vi "Data Logger Open Config.vi"(8 "error in":errorcluster, 10 "Cluster":T1, 11 "Path":path) -> (0 "error out":errorcluster)   [LabVIEW 2014]
uses:
  TypeDef/Datalogger_State_OpenConfigFile.ctl
  <vilib>/Utility/config.llb/Read Key (String).vi
  <vilib>/Utility/config.llb/Read Key (U32).vi
  <vilib>/Utility/config.llb/Read Key (Path).vi
  <vilib>/Utility/config.llb/Read Key (Boolean).vi
  <vilib>/Utility/config.llb/NI_LVConfig.lvlib
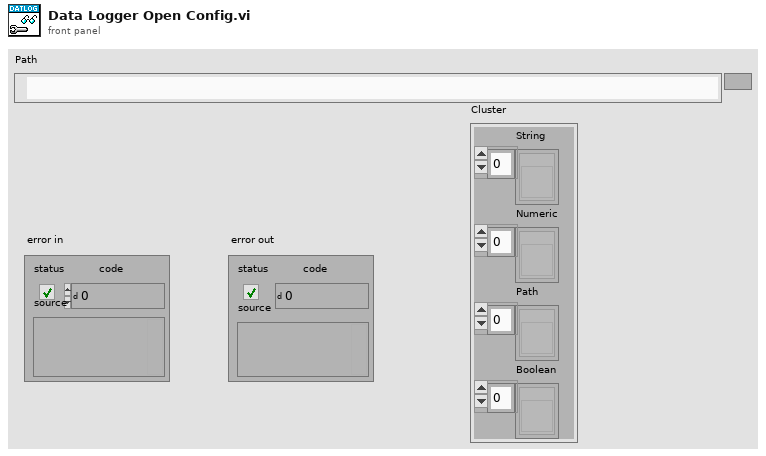
[diagram p1: front panel]
types:
  T1 = cluster{"String":refnum<vi>[], "Numeric":refnum<vi>[], "Path":refnum<vi>[], "Boolean":refnum<vi>[]}
  T2 = typedef "Datalogger_State_OpenConfigFile.ctl" = enum16{"Check config file?", "Open File", "Item 1", "Item 2", "Item 3", "Item 4", "Close File"}
  T3 = typedef "NI_LVConfig.lvlib/Config Data RefNum.ctl" = refnum<k1>
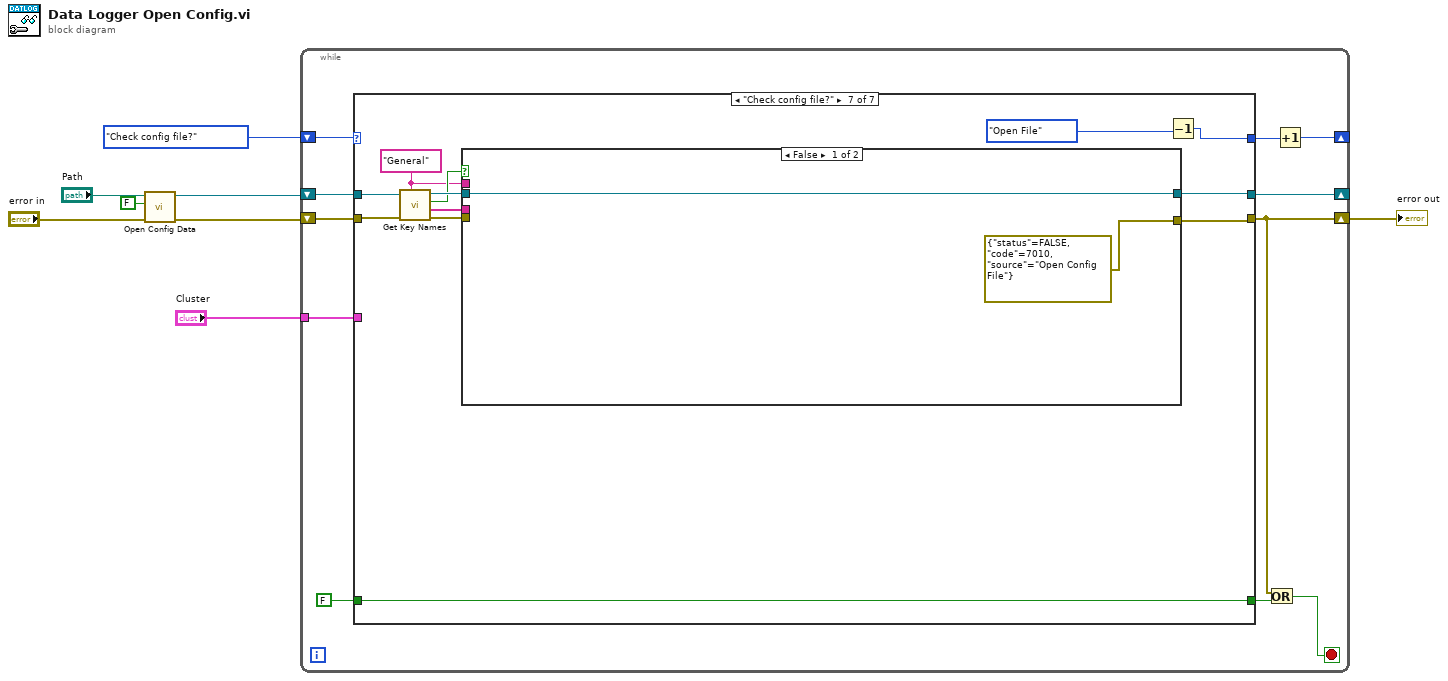
[diagram p0: block diagram]
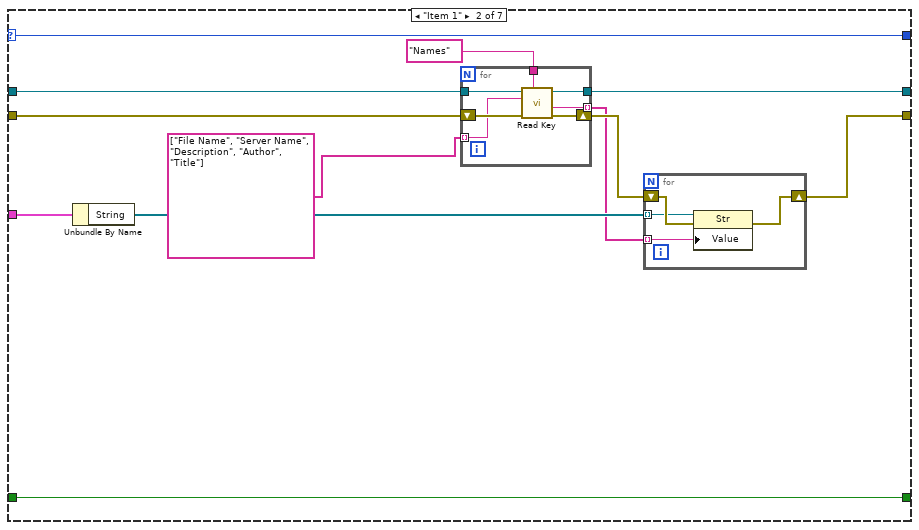
[diagram p3: hidden frame]
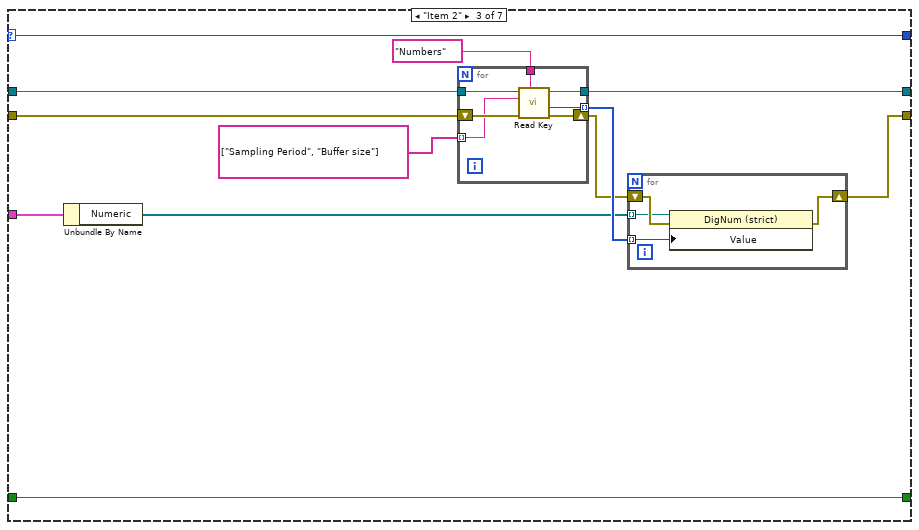
[diagram p4: hidden frame]
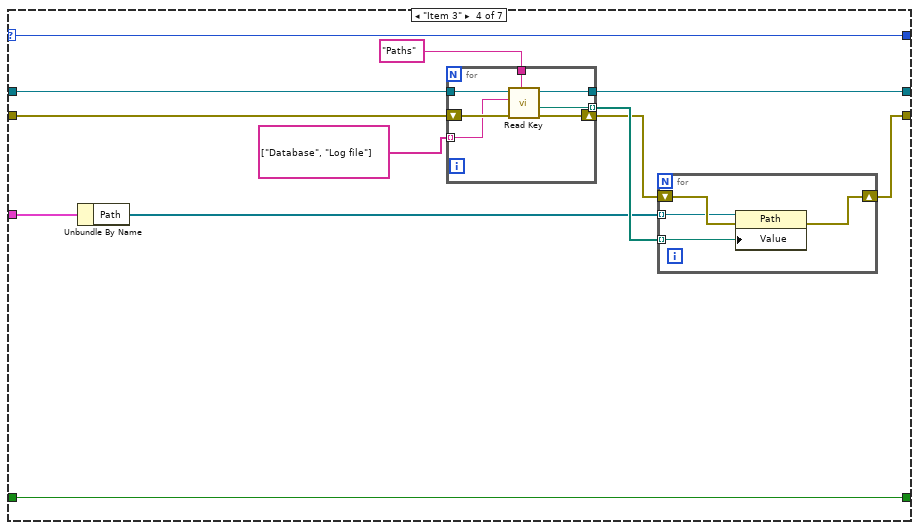
[diagram p5: hidden frame]
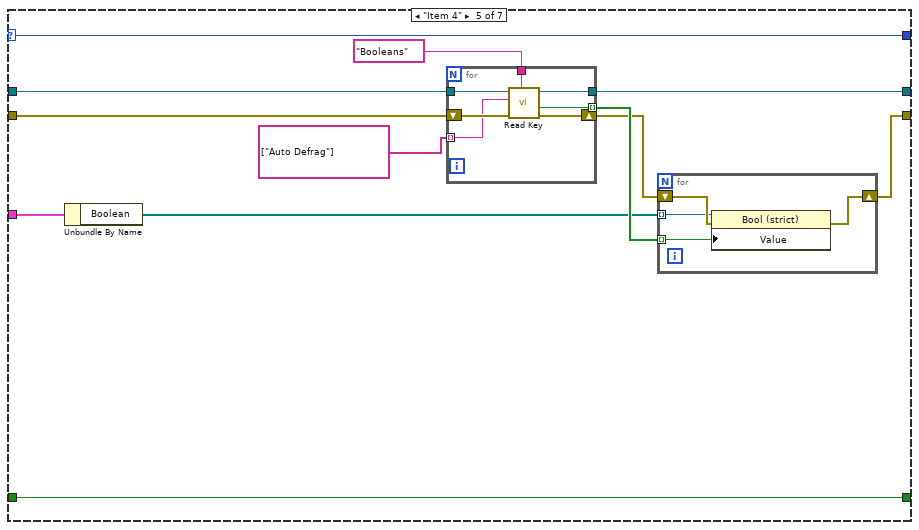
[diagram p6: hidden frame]
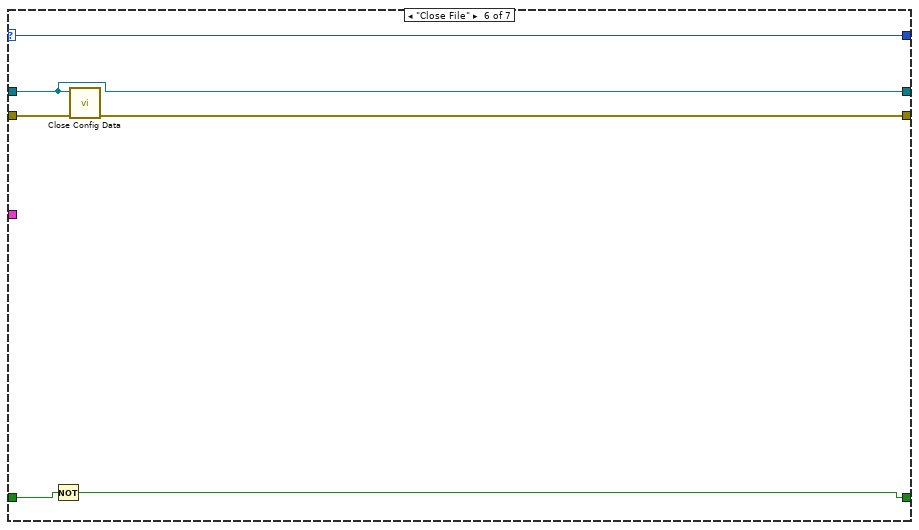
[diagram p7: hidden frame]
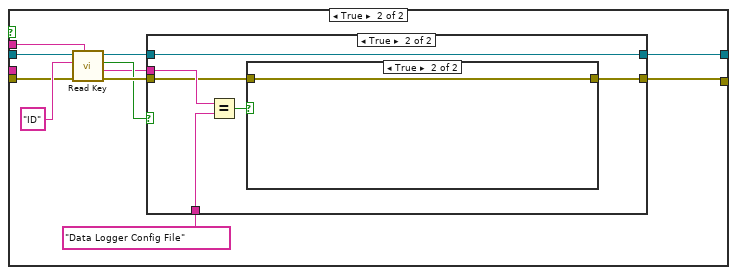
[diagram p8: hidden frame]
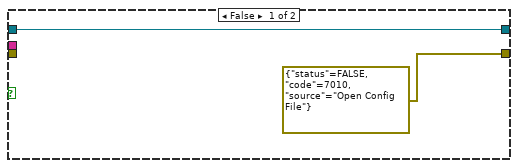
[diagram p9: hidden frame]
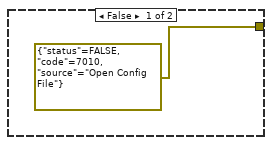
[diagram p10: hidden frame]
diagram:
  n1 = call <vilib>:"Open Config Data.vi"("error in (no error)"="error in", "create file if necessary (T)"=FALSE, "configuration file path"="Path") -> ("error out"=w6:errorcluster, "refnum"=w2:T3)  [unwired: 6 in, 1 out]
  n2 = while {
    shift-right: [w14] -> _
    shift-left: Datalogger_State_OpenConfigFile."Check config file?" -> [w19]
    tunnel: "Cluster" -> [w18]
    shift-right: [w9] -> w7
    shift-left: w6 -> [w17]
    shift-right: [w13] -> _
    shift-left: w2 -> [w16]
    stop <- w10 stop-if-true
    n3 = case shown="\"Check config file?\"" w19 {
      selector: w19 -> [w23 w35 w58 w81 w104 w118 _]
      tunnel: w18 -> [_ w34 w57 w80 w103 _ _]
      tunnel: [w23 w35 w58 w81 w104 w118 w122] -> w15
      tunnel: w17 -> [w21 w29 w50 w74 w97 w121 w130]
      tunnel: [w21 w25 w48 w71 w94 w120 w132] -> w9
      tunnel: [w20 w32 w55 w78 w101 w119 w124] -> w13
      tunnel: w16 -> [w20 w33 w56 w79 w102 w119 w131]
      tunnel: [w22 w30 w53 w76 w99 w116 w133] -> w11
      tunnel: FALSE -> [w22 w30 w53 w76 w99 w117 w133]
      frame "Open File", Default {
        # "Nothing for General to be done here"
      }
      frame "Item 1" {
        n4 = Unbundle By Name(w34) -> ("String"=w28:refnum<vi>[])
        n5 = for {
          tunnel: "Names" ("section") -> [w46]
          tunnel: w33 -> [w45]
          shift-right: [w43] -> w27
          shift-left: w29 -> [w44]
          tunnel: string[] ["File Name", "Server Name", "Description", "Author", "Title"] -> [w42] mode=indexing
          tunnel: [w41] -> w32
          tunnel: [w40] -> w26 mode=indexing
          n6 = call-poly <vilib>:"Read Key.vi"("section"=w46, "error in (no error)"=w44, "key"=w42, "refnum"=w45) -> ("error out"=w43:errorcluster, "value"=w40:string, "refnum out"=w41:T3)  [unwired: 4 in, 1 out]
        }
        n7 = for {
          shift-right: [w38] -> w25
          shift-left: w27 -> [w39]
          tunnel: w28 -> [w37] mode=indexing
          tunnel: w26 -> [w36] mode=indexing
          n8 = property class="Str"(reference=w37, error in=w39, "Value"=w36) -> (error out=w38:errorcluster)  [unwired: 1 out]
        }
      }
      frame "Item 2" {
        n9 = Unbundle By Name(w57) -> ("Numeric"=w51:refnum<vi>[])
        n10 = for {
          tunnel: "Numbers" ("section") -> [w69]
          tunnel: w56 -> [w68]
          shift-right: [w66] -> w49
          shift-left: w50 -> [w67]
          tunnel: string[] ["Sampling Period", "Buffer size"] -> [w65] mode=indexing
          tunnel: [w64] -> w55
          tunnel: [w63] -> w52 mode=indexing
          n11 = call-poly <vilib>:"Read Key.vi"("section"=w69, "error in (no error)"=w67, "key"=w65, "refnum"=w68) -> ("error out"=w66:errorcluster, "value"=w63:u32, "refnum out"=w64:T3)  [unwired: 4 in, 1 out]
        }
        n12 = for {
          shift-right: [w61] -> w48
          shift-left: w49 -> [w62]
          tunnel: w52 -> [w60] mode=indexing
          tunnel: w51 -> [w59] mode=indexing
          n13 = property class="DigNum (strict)"(reference=w59, error in=w62, "Value"=w60) -> (error out=w61:errorcluster)  [unwired: 1 out]
        }
      }
      frame "Item 3" {
        n14 = Unbundle By Name(w80) -> ("Path"=w73:refnum<vi>[])
        n15 = for {
          tunnel: "Paths" ("section") -> [w92]
          tunnel: w79 -> [w91]
          shift-right: [w89] -> w72
          shift-left: w74 -> [w90]
          tunnel: string[] ["Database", "Log file"] -> [w88] mode=indexing
          tunnel: [w87] -> w78
          tunnel: [w86] -> w75 mode=indexing
          n16 = call-poly <vilib>:"Read Key.vi"("section"=w92, "error in (no error)"=w90, "key"=w88, "refnum"=w91) -> ("error out"=w89:errorcluster, "value"=w86:path, "refnum out"=w87:T3)  [unwired: 4 in, 1 out]
        }
        n17 = for {
          shift-right: [w84] -> w71
          shift-left: w72 -> [w85]
          tunnel: w75 -> [w83] mode=indexing
          tunnel: w73 -> [w82] mode=indexing
          n18 = property class="Path"(reference=w82, error in=w85, "Value"=w83) -> (error out=w84:errorcluster)  [unwired: 1 out]
        }
      }
      frame "Item 4" {
        n19 = Unbundle By Name(w103) -> ("Boolean"=w96:refnum<vi>[])
        n20 = for {
          tunnel: "Booleans" ("section") -> [w115]
          tunnel: w102 -> [w114]
          shift-right: [w112] -> w95
          shift-left: w97 -> [w113]
          tunnel: string[] ["Auto Defrag"] -> [w111] mode=indexing
          tunnel: [w110] -> w101
          tunnel: [w109] -> w98 mode=indexing
          n21 = call-poly <vilib>:"Read Key.vi"("section"=w115, "error in (no error)"=w113, "key"=w111, "refnum"=w114) -> ("error out"=w112:errorcluster, "value"=w109:bool, "refnum out"=w110:T3)  [unwired: 4 in, 1 out]
        }
        n22 = for {
          shift-right: [w107] -> w94
          shift-left: w95 -> [w108]
          tunnel: w98 -> [w106] mode=indexing
          tunnel: w96 -> [w105] mode=indexing
          n23 = property class="Bool (strict)"(reference=w105, error in=w108, "Value"=w106) -> (error out=w107:errorcluster)  [unwired: 1 out]
        }
      }
      frame "Close File" {
        n24 = Not(x=w117) -> (.not. x?=w116:bool)
        n25 = call <vilib>:"Close Config Data.vi"("error in (no error)"=w121, "refnum"=w119) -> ("error out"=w120:errorcluster)  [unwired: 8 in, 1 out]
      }
      frame "Check config file?" {
        w125 = "General"
        n26 = call <vilib>:"Get Key Names.vi"("section"=w125, "error in (no error)"=w130, "refnum"=w131) -> ("error out"=w126:errorcluster, "key names"=w127:string[], "section exists?"=w128:bool, "refnum out"=w129:T3)  [unwired: 5 in]
        n27 = case shown="False" w128 {
          tunnel: [errorcluster {"status"=FALSE, "code"=7010, "source"="Open Config File"} ("error constant") w137] -> w132
          tunnel: w129 -> [w134 w146]
          tunnel: w127 -> [_ _]
          tunnel: w126 -> [_ w143]
          tunnel: w125 -> [_ w145]
          tunnel: [w134 w136] -> w124
          frame False {
          }
          frame True {
            n28 = call-poly <vilib>:"Read Key.vi"("section"=w145, "error in (no error)"=w143, "key"="ID" ("section"), "refnum"=w146) -> ("error out"=w141:errorcluster, "value"=w139:string, "found?"=w140:bool, "refnum out"=w142:T3)  [unwired: 4 in]
            n29 = case shown="True" w140 {
              tunnel: w142 -> [w148 w154]
              tunnel: [w148 w154] -> w136
              tunnel: w141 -> [_ w150]
              tunnel: w139 -> [_ w153]
              tunnel: "Data Logger Config File" ("section") -> [_ w152]
              tunnel: [errorcluster {"status"=FALSE, "code"=7010, "source"="Open Config File"} ("error constant") w149] -> w137
              frame False {
              }
              frame True {
                n30 = Equal?(x=w153, y=w152) -> (x = y?=w151:bool)
                n31 = case shown="True" w151 {
                  tunnel: w150 -> [_ w156]
                  tunnel: [errorcluster {"status"=FALSE, "code"=7010, "source"="Open Config File"} ("error constant") w156] -> w149
                  frame False {
                  }
                  frame True {
                  }
                }
              }
            }
          }
        }
        n32 = Decrement(x=Datalogger_State_OpenConfigFile."Open File") -> (x-1=w122:T2)
      }
    }
    n33 = Or(x=w9, y=w11) -> (x .or. y?=w10:bool)
    n34 = Increment(x=w15) -> (x+1=w14:T2)
  }
  "error out" <- w7
